vi "Spindexer_Set.vi"   [LabVIEW 2019]
uses:
  Globals/Spindexer_Globals.vi
  Spindexer_mode.ctl
types:
  T1 = typedef "Spindexer_mode.ctl" = enum16{"No-Op", "Sensing", "Intaking", "Firing(Speed Control)", "Manual"}
  T2 = typedef "Spindexer_Cluster.ctl" = cluster{"Throttle":dbl, "Fire?":bool, "Intake recently moved?":bool, "Mode":T1, "Sensor in position? ":bool}
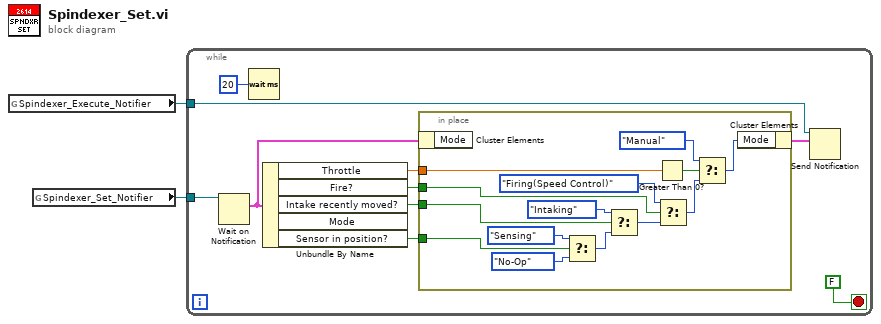
[diagram p0: block diagram]
diagram:
  n1 = global read "Spindexer_Globals.vi" "Spindexer_Execute_Notifier"() -> (w1:refnum<notifier>)
  n2 = global read "Spindexer_Globals.vi" "Spindexer_Set_Notifier"() -> (w2:refnum<notifier>)
  n3 = while {
    tunnel: w2 -> [w10]
    tunnel: w1 -> [w9]
    stop <- FALSE stop-if-true
    n4 = Wait on Notification(notifier=w10) -> (notification=w7:T2)  [unwired: 3 in, 3 out]
    n5 = Wait (ms)(milliseconds to wait=u32 20 ("millisecond timer value")) -> ()  [unwired: 1 out]
    n6 = Unbundle By Name(w7) -> ("Throttle"=w3:dbl, "Fire?"=w4:bool, "Intake recently moved?"=w5:bool, "Sensor in position?"=w6:bool)  [unwired: 1 out]
    n7 = in-place {
      in-place-border: w6 -> [w26]
      in-place-border: w5 -> [w23]
      in-place-border: w4 -> [w20]
      in-place-border: w3 -> [w14]
      n8 = in-place-cluster #1(w7) -> ()  [unwired: 1 out]
      n9 = Select(t=Spindexer_mode."Sensing" ("Mode"), s=w26, f=Spindexer_mode."No-Op" ("Mode")) -> (s? t:f=w22:T1)
      n10 = Select(t=Spindexer_mode."Intaking" ("Mode"), s=w23, f=w22) -> (s? t:f=w19:T1)
      n11 = Greater Than 0?(x=w14) -> (x > 0?=w13:bool)
      n12 = Select(t=Spindexer_mode."Firing(Speed Control)" ("Mode"), s=w20, f=w19) -> (s? t:f=w16:T1)
      n13 = Select(t=Spindexer_mode."Manual" ("Mode"), s=w13, f=w16) -> (s? t:f=w17:T1)
      n14 = in-place-cluster #1("Mode"=w17) -> (w8:T2)
    }
    n15 = Send Notification(notification=w8, notifier=w9) -> ()  [unwired: 1 in, 2 out]
  }
